vi "Generate Unique ID.vi"(8 "error in (no error)":errorcluster, 11 "Linked List in":refnum<class "Linked List.lvclass">) -> (0 "error out":errorcluster, 2 "ID":string, 3 "Linked List out":refnum<class "Linked List.lvclass">)   [LabVIEW 2020, in "Linked Lists.lvlib" / "Linked List.lvclass"]
uses:
  <vilib>/gpm_packages/@cs/linked-list/Source/Linked List/Linked List/Linked List.lvclass
  <vilib>/gpm_packages/@cs/linked-list/Source/Linked List/Linked List/Linked List.lvclass/Linked List.ctl
  <vilib>/gpm_packages/@cs/lookup-table/Source/LookupTable/LookupTable.lvclass/LookupTable.ctl
  14d8632b-b3dd-4e54-92d2-d0c870543d30.vi
  <vilib>/gpm_packages/@cs/lookup-table/Source/LookupTable/Read Table Reference.vi
  14d8632b-b3dd-4e54-92d2-d0c870543d30.vi/9f5662a4-523d-4a96-8a6c-36f6820bf389.vi
  <vilib>/gpm_packages/@cs/lookup-table/Source/LookupTable/LookupTable.lvclass
  <vilib>/gpm_packages/@cs/linked-list/Source/String Manipulation/String Manipulation.lvlib
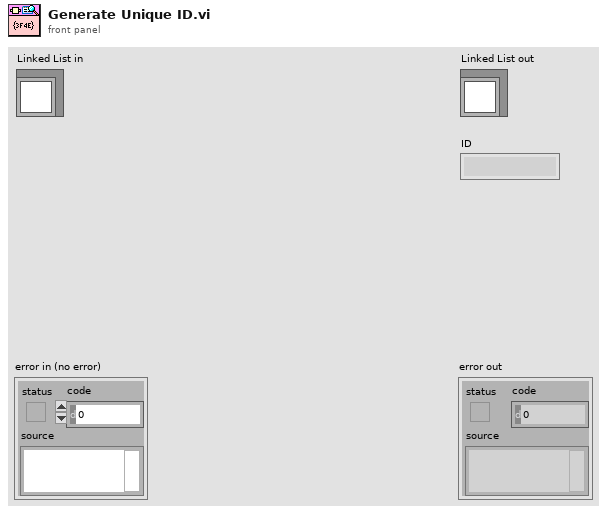
[diagram p1: front panel]
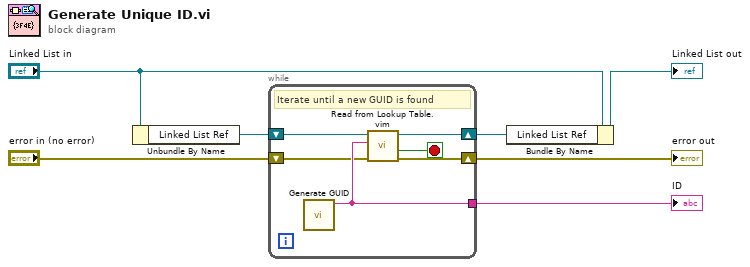
[diagram p0: block diagram]
diagram:
  n1 = Unbundle By Name("Linked List in") -> ("Linked List Ref"=w7:refnum<data-value>)
  n2 = while {
    shift-right: [w12] -> w6
    shift-left: w7 -> [w13]
    tunnel: [w10] -> w3
    shift-right: [w8] -> w1
    shift-left: "error in (no error)" -> [w9]
    stop <- w11 stop-if-true
    # "Iterate until a new GUID is found"
    n3 = call <vilib>:"Generate GUID.vi"() -> ("Hash"=w10:string)  [unwired: 10 in, 1 out]
    n4 = call "Read from Lookup Table.vim"("error in (no error)"=w9, "Item Name"=w10, "LookupTable Reference"=w13) -> ("error out"=w8:errorcluster, "Not Found?"=w11:bool, "LookupTable Reference Out"=w12:refnum<data-value>)  [unwired: 5 in, 1 out]
  }
  "error out" <- w1
  "ID" <- w3
  n5 = Bundle By Name(cluster="Linked List in", "Linked List Ref"=w6) -> (→"Linked List out":refnum<class "Linked List.lvclass">)
